vi "TestReadSignal.vi"() -> ()   [LabVIEW 2017]
uses:
  DataChannel.ctl
  DataFrontPanel.ctl
panel:
  in  "stop":bool=TRUE
  out "XY Graph":cluster{cluster{dbl, "Data":dbl}[]}[](graph)
  in  "Data points":i32=100
  in  "DataFrontPanel":T1=2 caption="Data channel" items=["Green", "Blue", "Yellow", "Orange"]
  in  "DataChannel":T2=2 caption="Data channel" items=["X", "Y", "R", "Theta", "IN1", "IN2", "IN3", "IN4", "OUT1", "OUT2", "XNoise", "YNoise", "Phase", "SineOut", "DCLevel", "IntRefFreq", "ExtRefFreq"]
  in  "VISA resource name":refnum<visa-resource-name>="USB0::0xB506::0x2000::002616::INSTR"
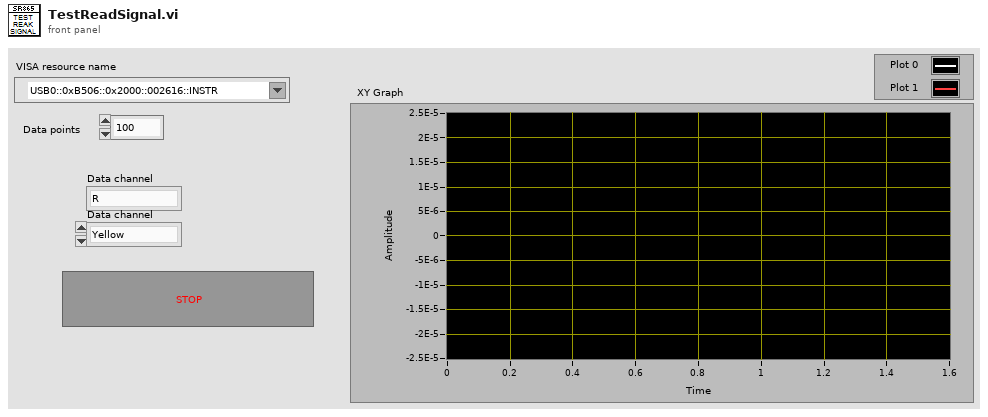
[diagram p1: front panel]
types:
  T1 = typedef "DataFrontPanel.ctl" = u16
  T2 = typedef "DataChannel.ctl" = u16
  T3 = typedef "SR865.ctl" = cluster{"VISA resource name":refnum<visa-resource-name>, "ReadWrite":T4}
  T4 = typedef "Semaphore RefNum" = refnum<k1>
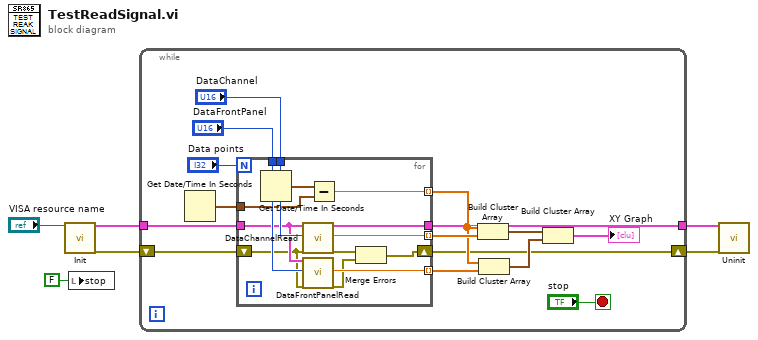
[diagram p0: block diagram]
diagram:
  n1 = call "Init.vi"("VISA resource name"="VISA resource name") -> ("SR865"=w4:T3, "error out"=w5:errorcluster)  [unwired: 17 in]
  n2 = local write "stop"(FALSE ("stop")) -> ()
  n3 = while {
    tunnel: w4 -> [w11]
    tunnel: [w10] -> w3
    shift-right: [w8] -> w2
    shift-left: w5 -> [w9]
    stop <- "stop" stop-if-true
    n4 = Get Date/Time In Seconds() -> (seconds since 1Jan1904=w18:timestamp)
    n5 = for {
      N: "Data points" -> [_]
      tunnel: "DataFrontPanel" -> [w34]
      tunnel: "DataChannel" -> [w33]
      tunnel: w18 -> [w22]
      tunnel: [w32] -> w17 mode=indexing
      tunnel: [w31] -> w15 mode=indexing
      tunnel: [w30] -> w16 mode=indexing
      tunnel: w11 -> [w29]
      tunnel: [w28] -> w10
      shift-right: [w25] -> w8
      shift-left: w9 -> [w26]
      n6 = Get Date/Time In Seconds() -> (seconds since 1Jan1904=w23:timestamp)
      n7 = call "DataChannelRead.vi"("SR865 in"=w29, "DataChannel"=w33, "error in"=w26) -> ("SR865 out"=w28:T3, "Signal"=w32:dbl, "error out"=w27:errorcluster)  [unwired: 14 in]
      n8 = call "DataFrontPanelRead.vi"("SR865 in"=w29, "DataFrontPanel"=w34, "error in"=w26) -> ("Data"=w31:dbl, "error out"=w24:errorcluster)  [unwired: 14 in, 1 out]
      n9 = Subtract(x=w23, y=w22) -> (x-y=w30:dbl)
      n10 = Merge Errors(w27, w24) -> (w25:errorcluster)
    }
    n11 = Build Cluster Array(w16, w17) -> (w14:cluster{dbl, "Signal":dbl}[])
    n12 = Build Cluster Array(w16, w15) -> (w12:cluster{dbl, "Data":dbl}[])
    n13 = Build Cluster Array(w14, w12) -> (→"XY Graph":cluster{cluster{dbl, "Data":dbl}[]}[])
  }
  n14 = call "Uninit.vi"("SR865 in"=w3, "error in"=w2) -> ()  [unwired: 17 in, 1 out]
